vi "Get Port.vi"(8 "error in (no error)":errorcluster, 10 "index":i32, 11 "Ports in":refnum<class "Ports.lvclass">) -> (0 "error out":errorcluster, 2 "Port":cluster{"String":string, "Array 2":bool[]}, 3 "Ports out":refnum<class "Ports.lvclass">)   [LabVIEW 2010, in "Ports.lvclass"]
uses:
  Ports.lvclass
  Ports.lvclass/Ports.ctl
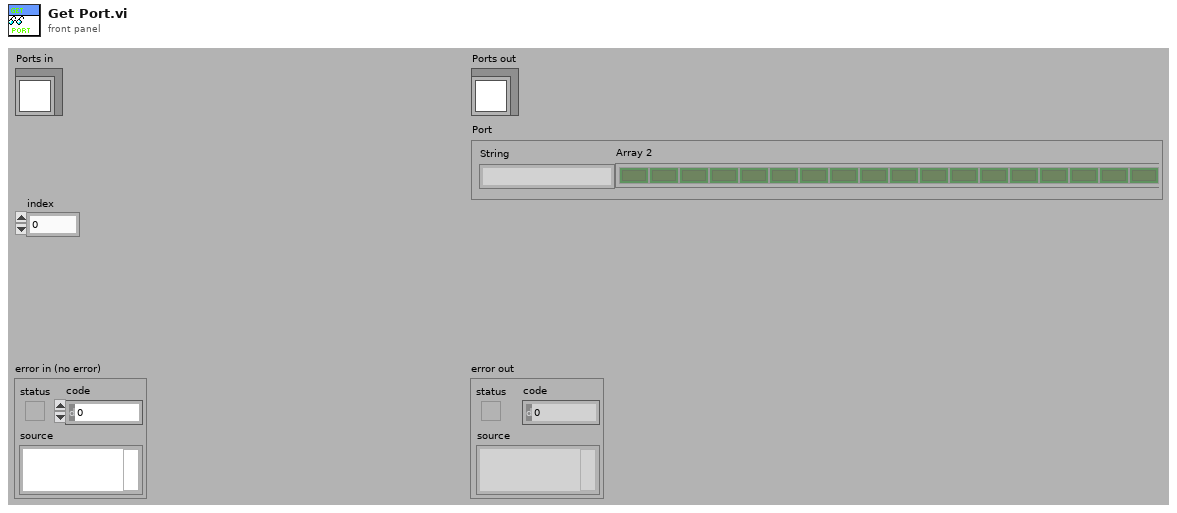
[diagram p1: front panel]
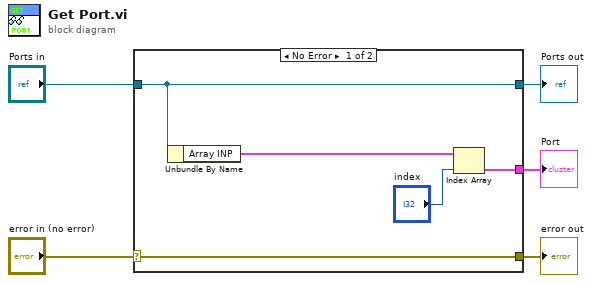
[diagram p0: block diagram]
diagram:
  n1 = case shown="No Error" "error in (no error)" {
    selector: "error in (no error)" -> [w10 w11]
    tunnel: [w10 w11] -> w4
    tunnel: [w9 w12] -> w2
    tunnel: "Ports in" -> [w9 w12]
    tunnel: [w6 _] -> w1
    frame No Error {
      n2 = Unbundle By Name(w9) -> ("Array INP"=w8:cluster{"String":string, "Array 2":bool[]}[])
      n3 = Index Array(array=w8, index="index") -> (element=w6:cluster{"String":string, "Array 2":bool[]})
    }
    frame Error {
    }
  }
  "error out" <- w4
  "Ports out" <- w2
  "Port" <- w1
